vi "Multichannel Recording0.3.vi"() -> ()   [LabVIEW 2014]
uses:
  Enum State Typedef.ctl
  <vilib>/Utility/error.llb/DialogType.ctl
  <vilib>/_DAQmxBase/Internals/DAQmxBase Create Channel (AI-Voltage-Basic).vi
  <vilib>/_DAQmxBase/Internals/DAQmxBase Timing (Sample Clock).vi
  <vilib>/_DAQmxBase/Internals/DAQmxBase Read (Analog 2D DBL NChan NSamp).vi
panel:
  in  "Use Channel 0":bool caption="In Use?"
  in  "Use Channel 2":bool caption="In Use?"
  in  "Use Channel 3":bool caption="In Use?"
  in  "Use Channel 1":bool caption="In Use?"
  in  "Open Button":bool
  in  "Tab Control":T1(tab)
  in  "Amplifier Channel 0":T2 {"Amplifier Model" items=["Select a Model", "AM 1700", "BMA 200"]}
  out "Channel 0 Chart":waveform(dbl)(graph)
  in  "User Data Channel 0":T3
  out "Channel 1 Chart":waveform(dbl)(graph)
  in  "User Data Channel 1":T3
  in  "Amplifier Channel 1":T2 {"Amplifier Model" items=["Select a Model", "AM 1700", "BMA 200"]}
  out "Channel 2 Chart":waveform(dbl)(graph)
  in  "User Data Channel 2":T3
  in  "Amplifier Channel 2":T2 {"Amplifier Model" items=["Select a Model", "AM 1700", "BMA 200"]}
  out "Channel 3 Chart":waveform(dbl)(graph)
  in  "User Data Channel 3":T3
  in  "Amplifier Channel 3":T2 {"Amplifier Model" items=["Select a Model", "AM 1700", "BMA 200"]}
  out "Overview Chart":waveform(dbl)[](graph)
  in  "Stop Preview":bool
  in  "OK Button":bool
  out "State":T4
  in  "Clear Display":bool
  in  "Preview Button":bool
  out "Iterations Recorded":i32
  in  "Recording Time (seconds)":dbl
  in  "Sample Rate":i32=1000
  in  "Stop Button":bool
  out "Start Time hr/min":string
  out "Date mm/dd/yy":string
  in  "Exit Button":bool
  in  "Record Button":bool
  # "MSU EFISH Lab Multi-Channel Electronic Pulse Recorder"
  # "Must enter numbers into here before you start"
  # "Blue for On\nOrange for Off"
  # "DC"
  # "AC"
  # "Blue for AC and Orange for DC"
  # "Blue for On\nOrange for Off"
  # "DC"
  # "AC"
  # "Blue for AC and Orange for DC"
  # "Blue for On\nOrange for Off"
  # "DC"
  # "AC"
  # "Blue for AC and Orange for DC"
  # "Blue for On\nOrange for Off"
  # "DC"
  # "AC"
  # "Blue for AC and Orange for DC"
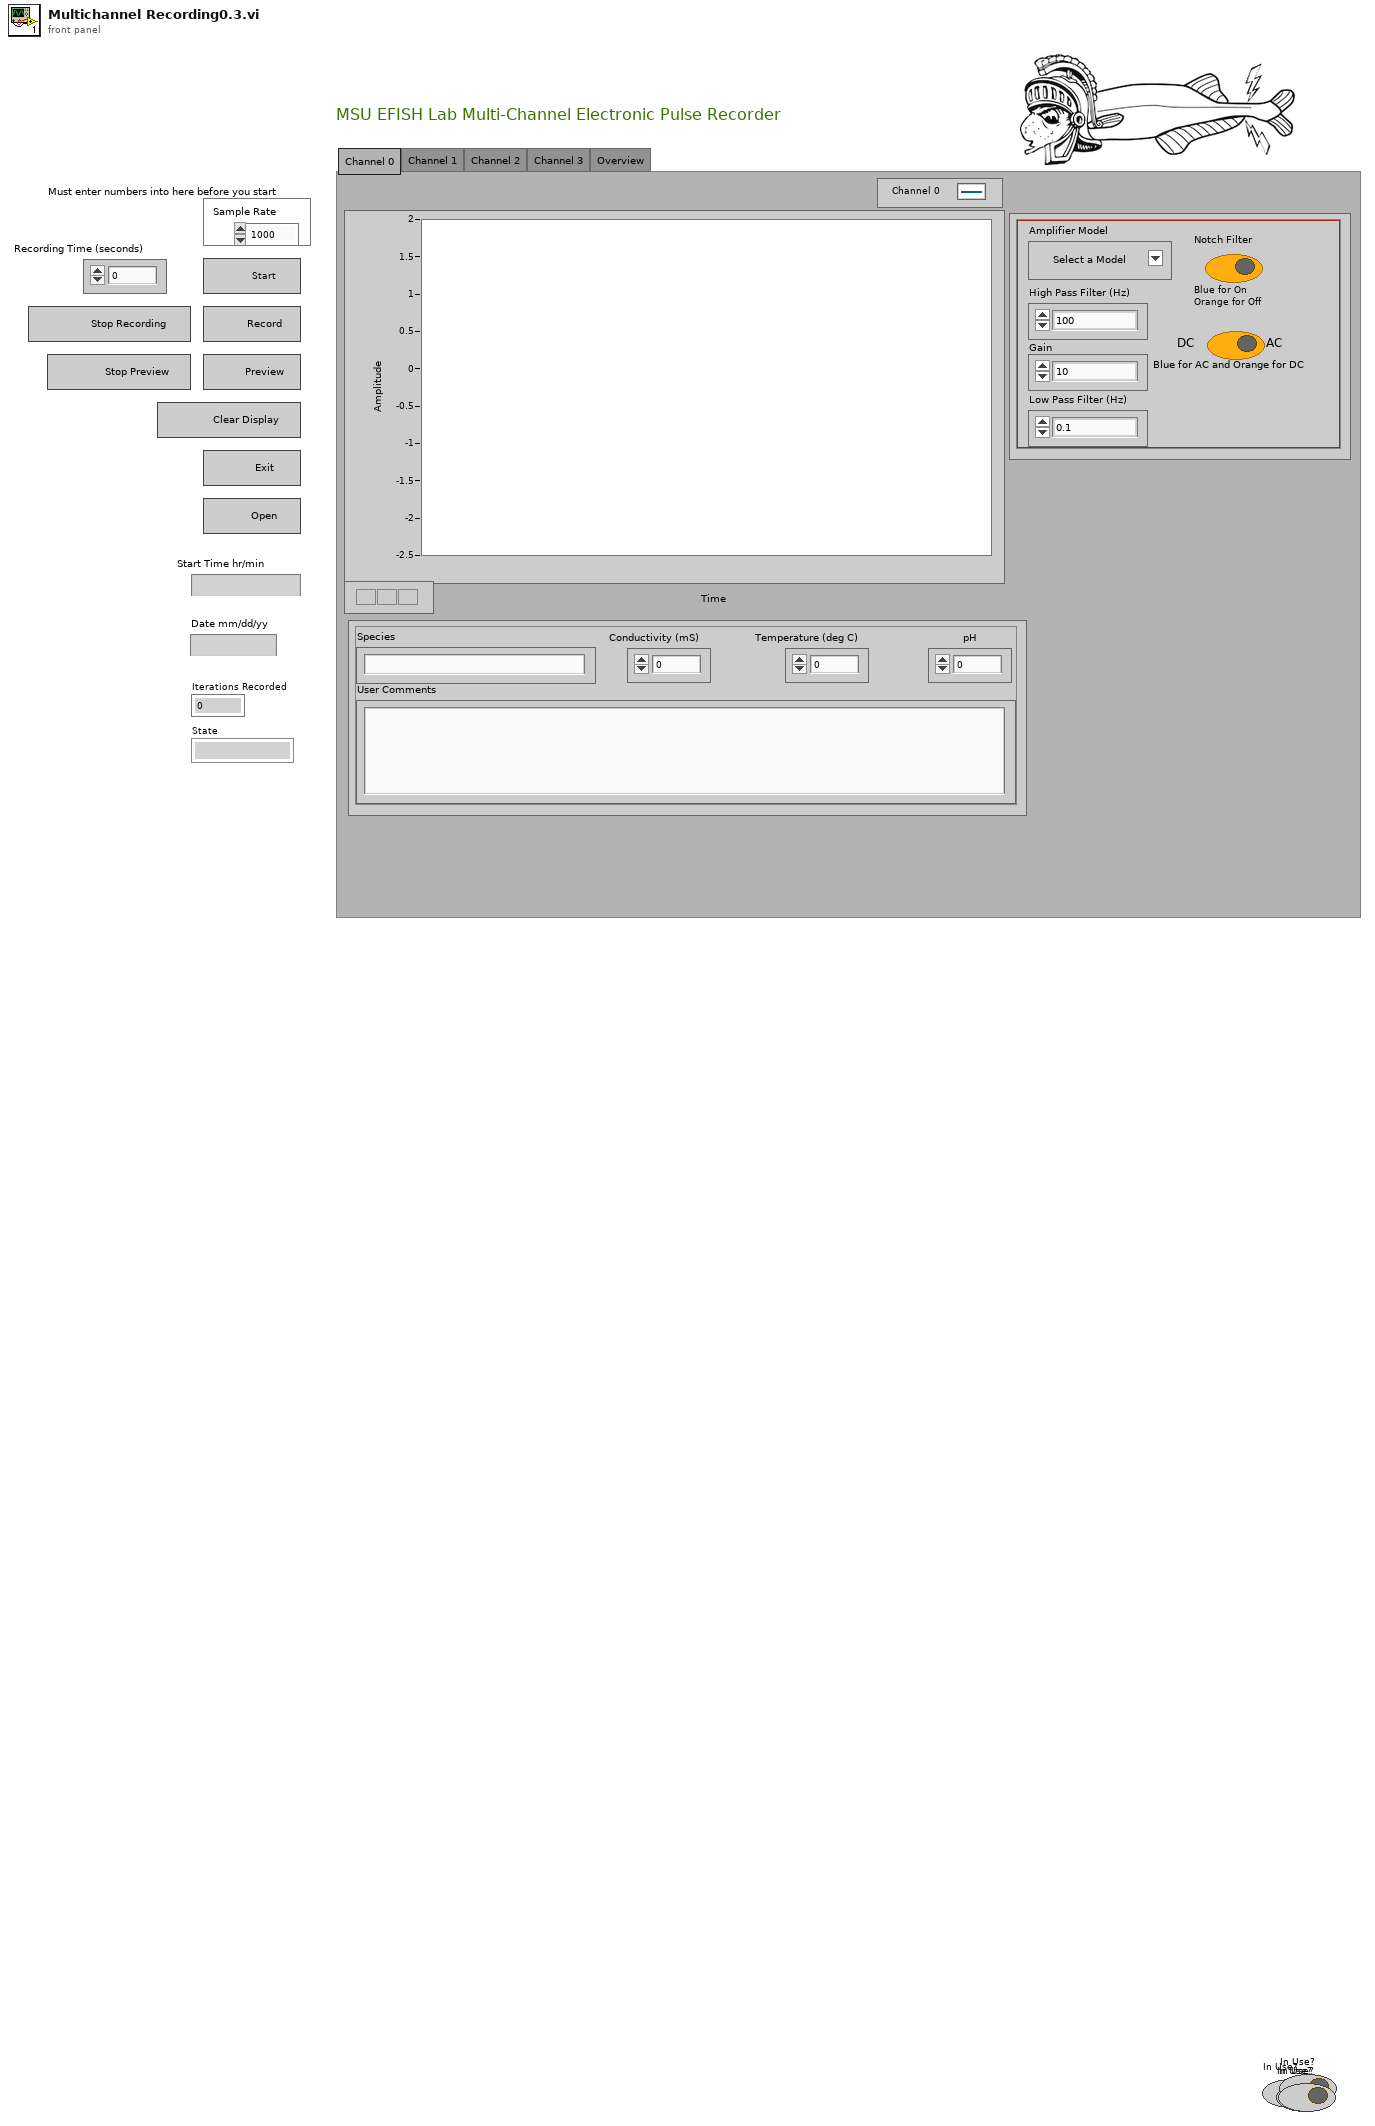
[diagram p1: front panel]
types:
  T1 = enum32{"Channel 0", "Channel 1", "Channel 2", "Channel 3", "Overview"}
  T2 = cluster{"Low Pass Filter (Hz)":enum16{"0.1", "1", "3", "10", "30", "100", "300"}, "Gain ":enum16{"10", "20", "50", "100", "200", "500", "1000", "2k", "5k", "10k", "20k", "50k"}, "High Pass Filter (Hz)":enum16{"100", "500", "1000", "3000", "5000", "10,000", "20,000", "30,000", "50,000"}, "Notch Filter":bool, "Amplifier Model":u16, "AC/DC Switch":bool}
  T3 = cluster{"pH":dbl, "Conductivity (mS)":dbl, "Temperature (deg C)":dbl, "User Comments":string, "Species":string}
  T4 = typedef "Enum State Typedef.ctl" = enum16{"", "Open FIle", "Beginning State", "Set the Sample Clock", "Prepreview Handling", "Clear Display", "Preview Data", "Stop", "Exit", "Record", "Create File"}
  T5 = cluster{"tdms file out":refnum<k34>, "tdms file out":refnum<k34>, "tdms file out":refnum<k34>, "tdms file out":refnum<k34>}
  T6 = enum8{"Enabled", "Disabled", "Disabled and Grayed Out"}
  T7 = typedef "DialogType.ctl" = u16
  T8 = enum16{"open", "open or create", "create or replace", "create", "open (read-only)"}
  T9 = cluster{"Use Channel 0":bool, "Use Channel 1":bool, "Use Channel 2":bool, "Use Channel 3":bool}
  T10 = cluster{"Waveform":waveform(dbl), "Waveform":waveform(dbl), "Waveform":waveform(dbl), "Waveform":waveform(dbl), waveform(dbl)[]}
  T11 = cluster{"Waveform":waveform(dbl), "Waveform":waveform(dbl), "Waveform":waveform(dbl), "Waveform":waveform(dbl)}
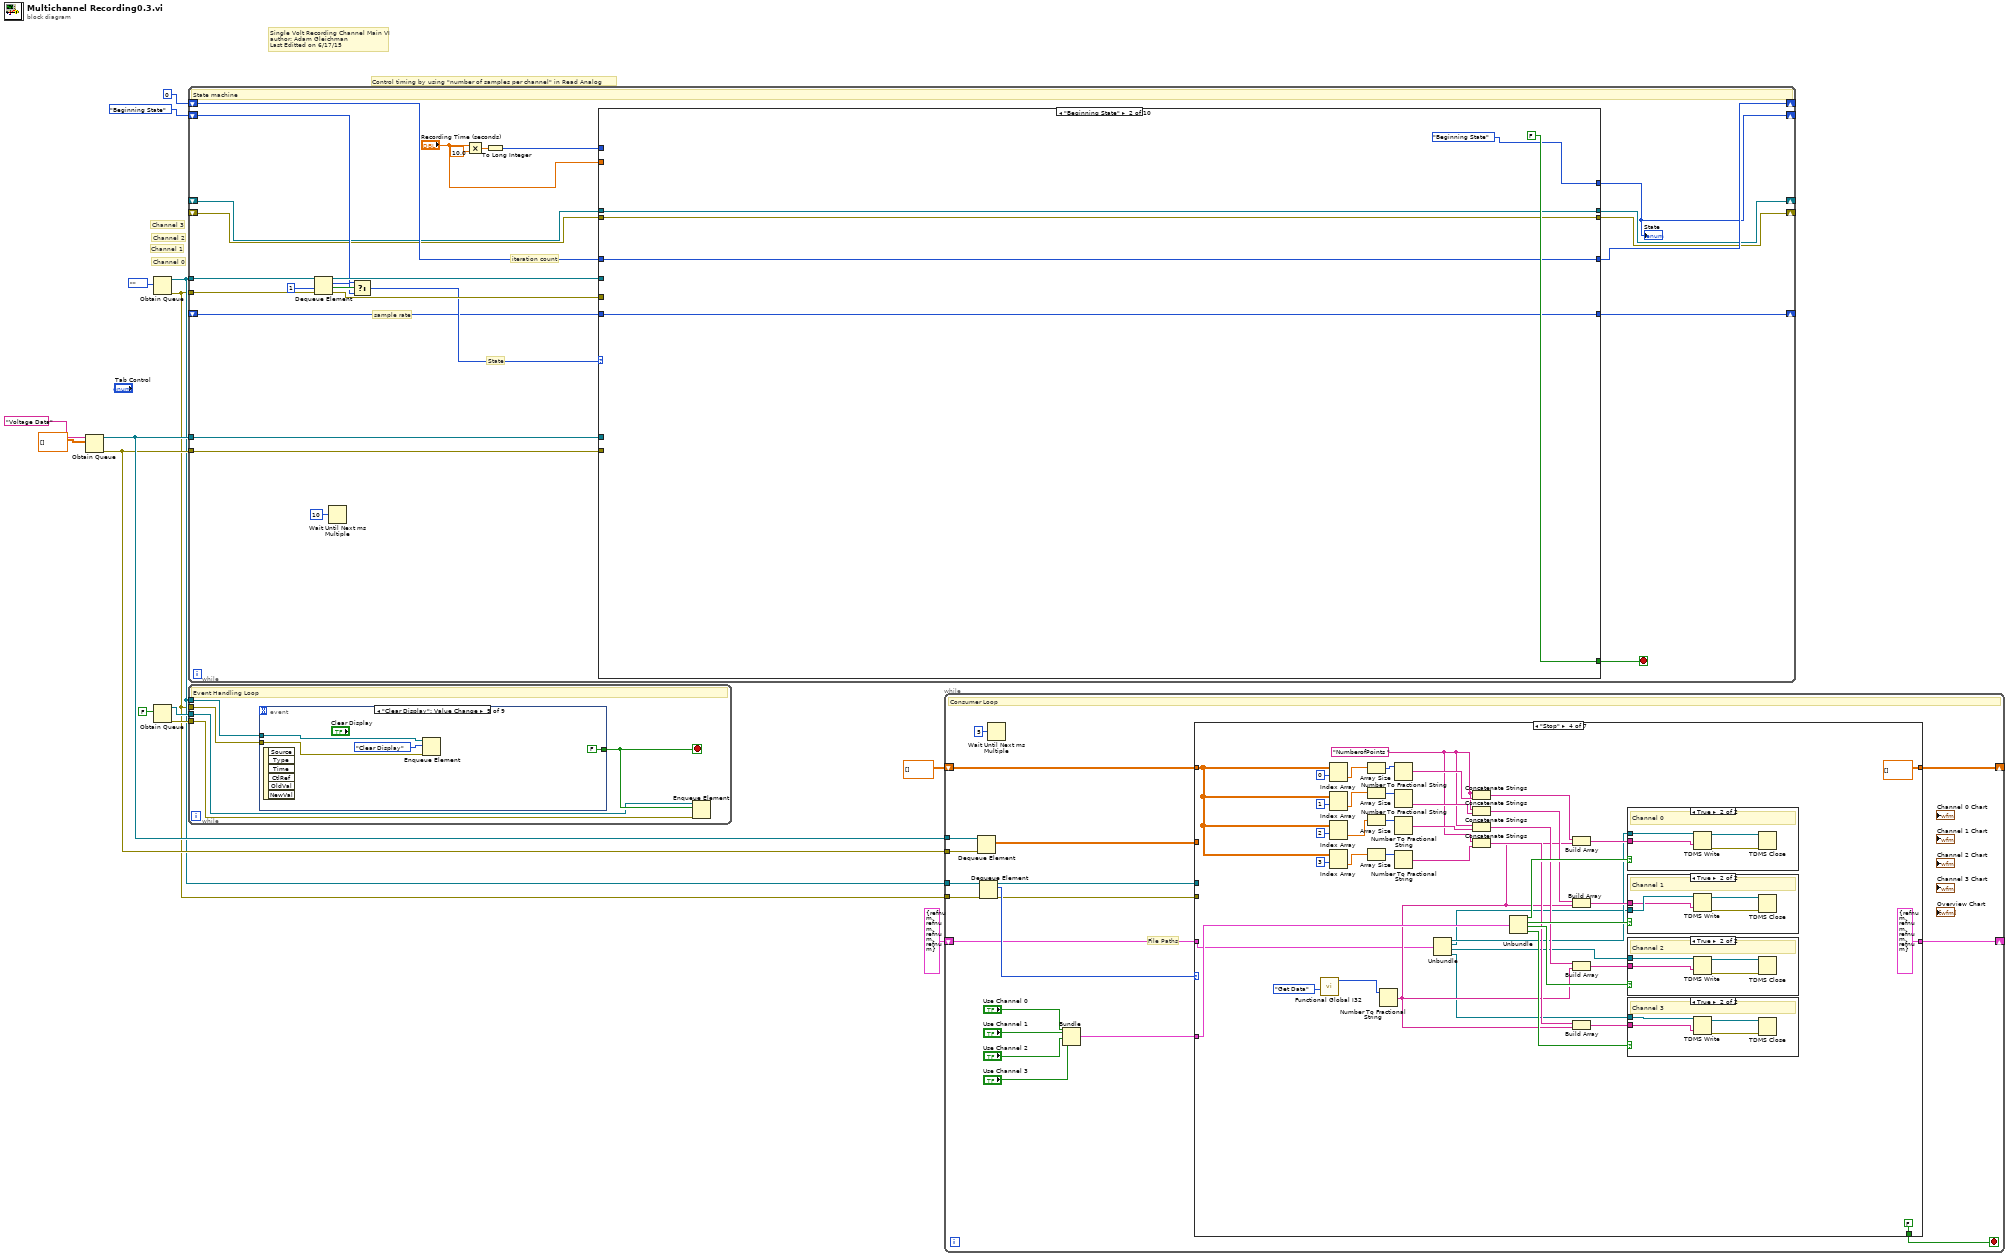
[diagram p0: block diagram]
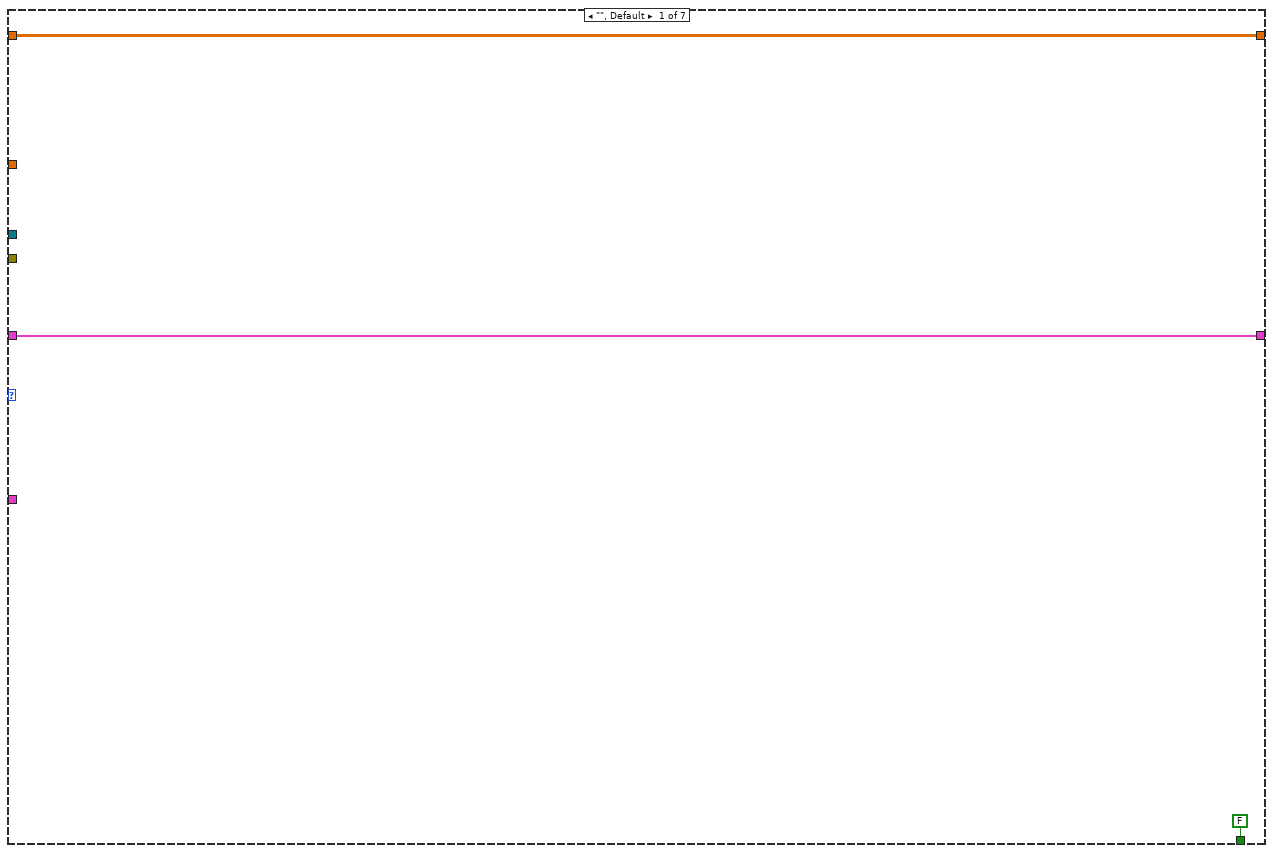
[diagram p2: hidden frame]
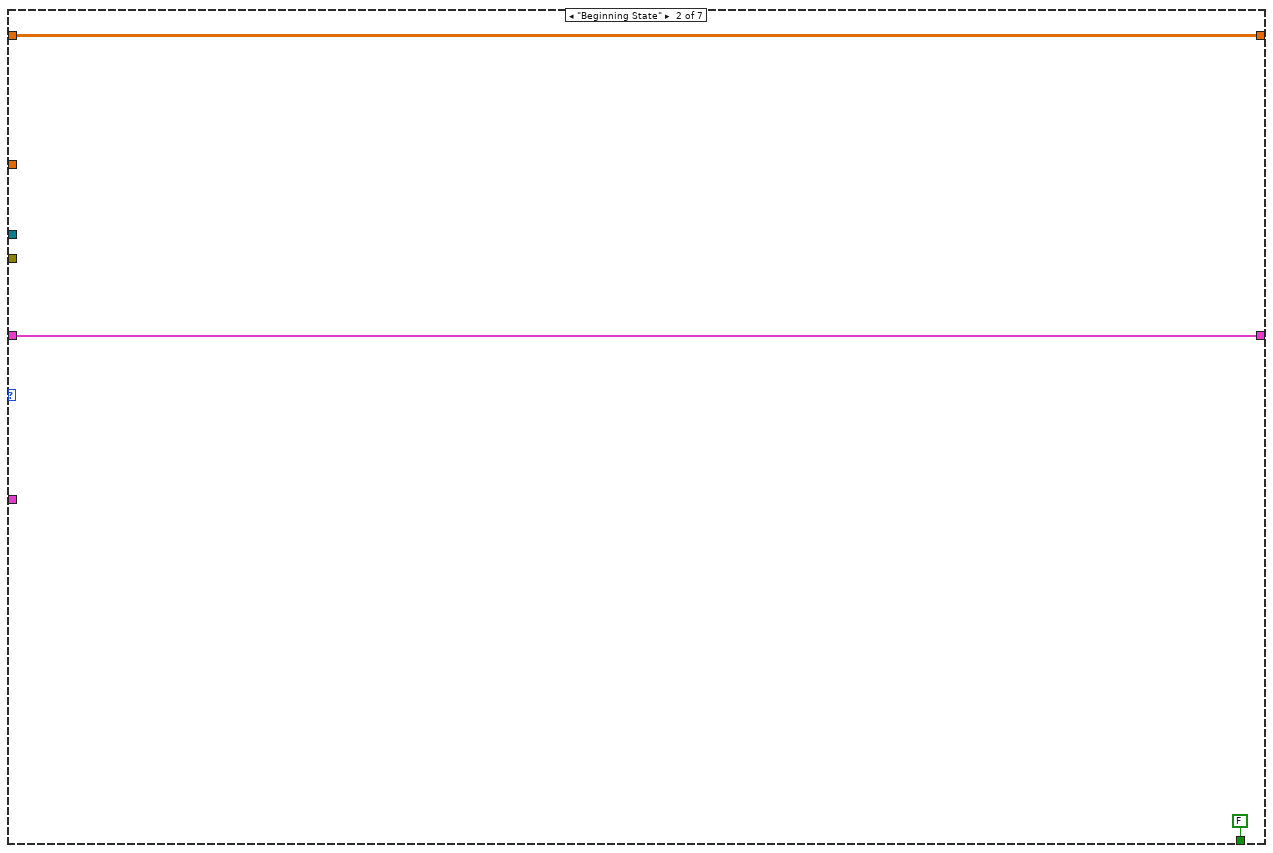
[diagram p3: hidden frame]
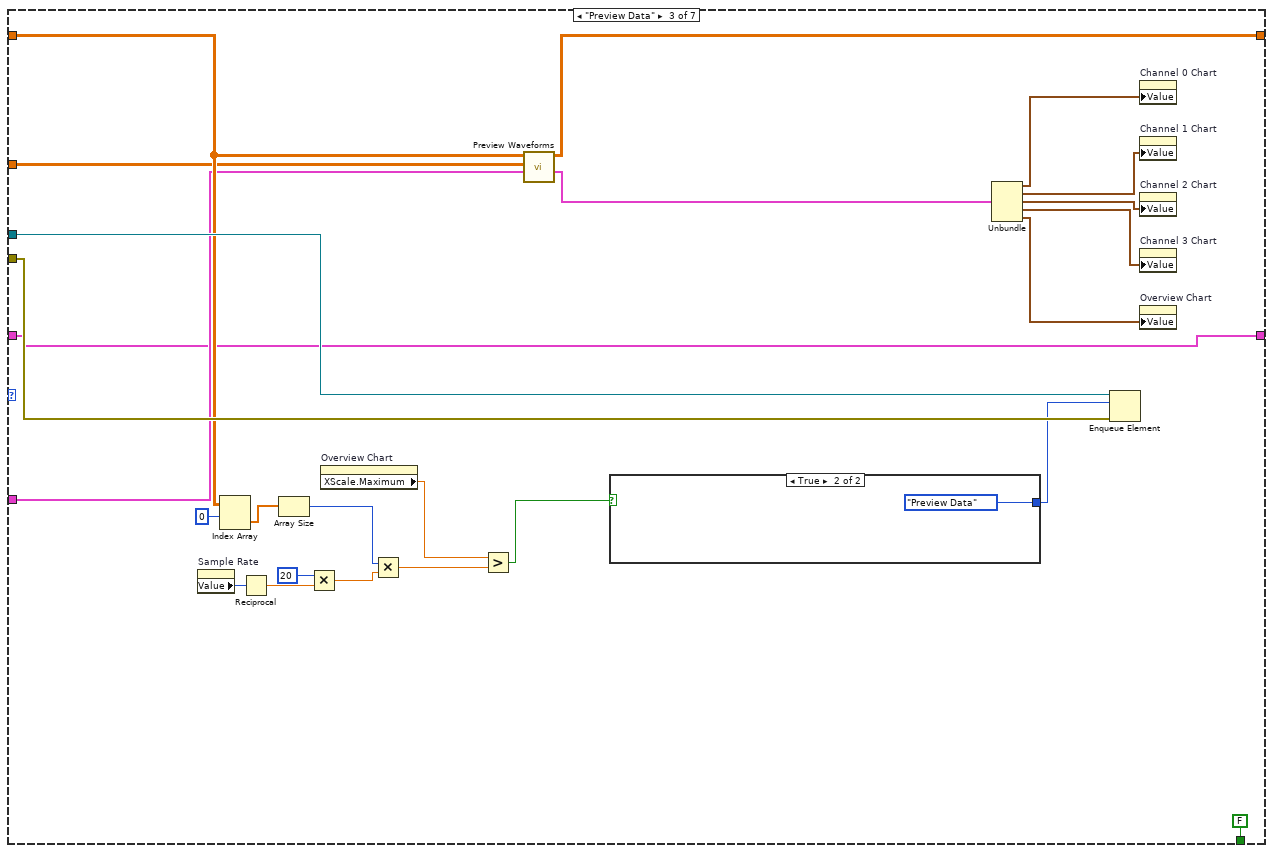
[diagram p4: hidden frame]
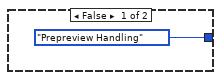
[diagram p5: hidden frame]
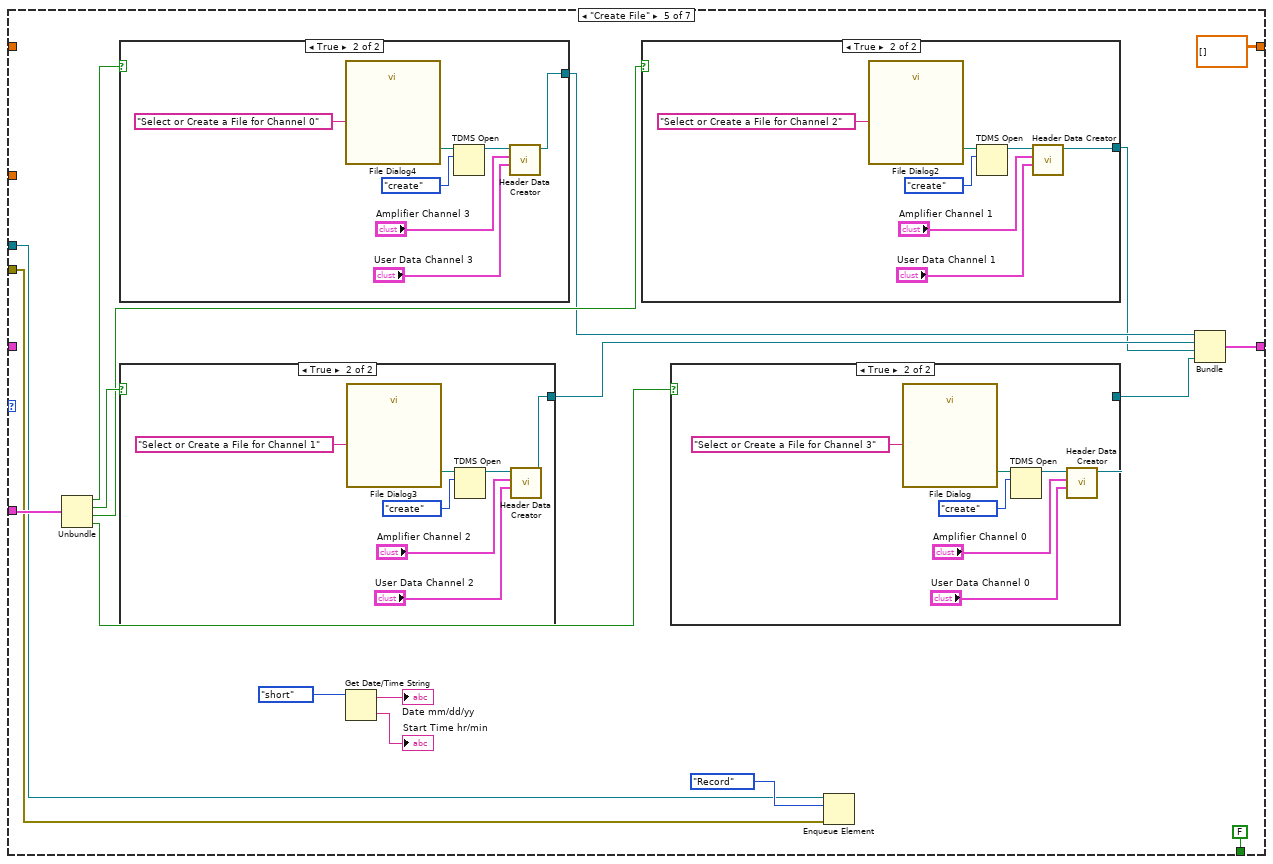
[diagram p10: hidden frame]
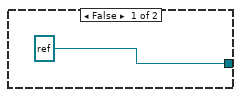
[diagram p11: hidden frame]
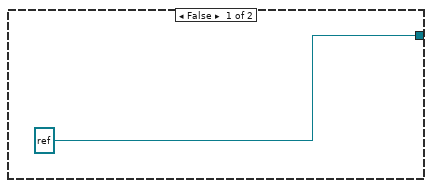
[diagram p12: hidden frame]
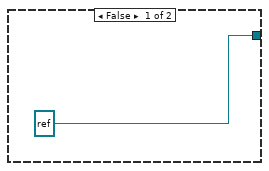
[diagram p13: hidden frame]
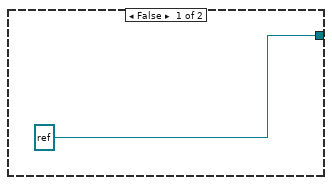
[diagram p14: hidden frame]
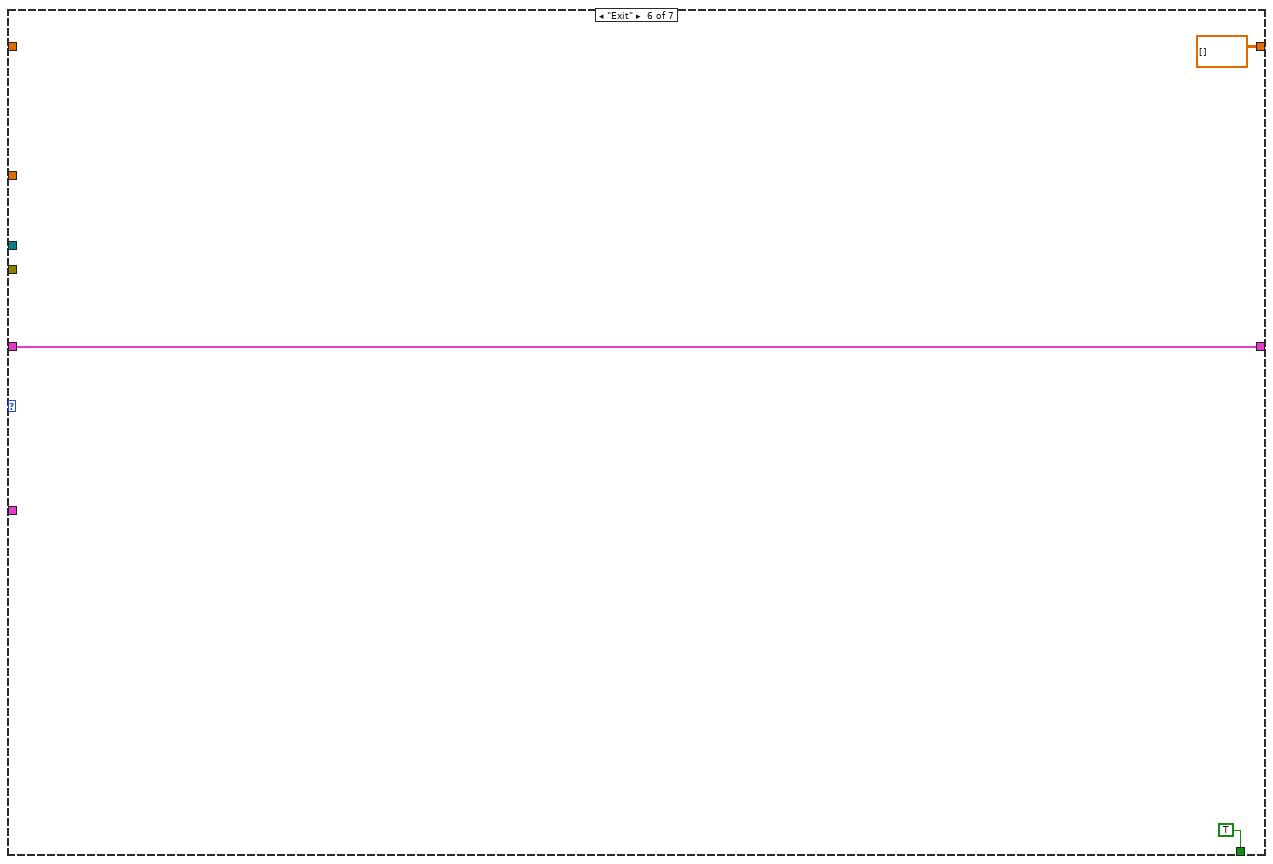
[diagram p15: hidden frame]
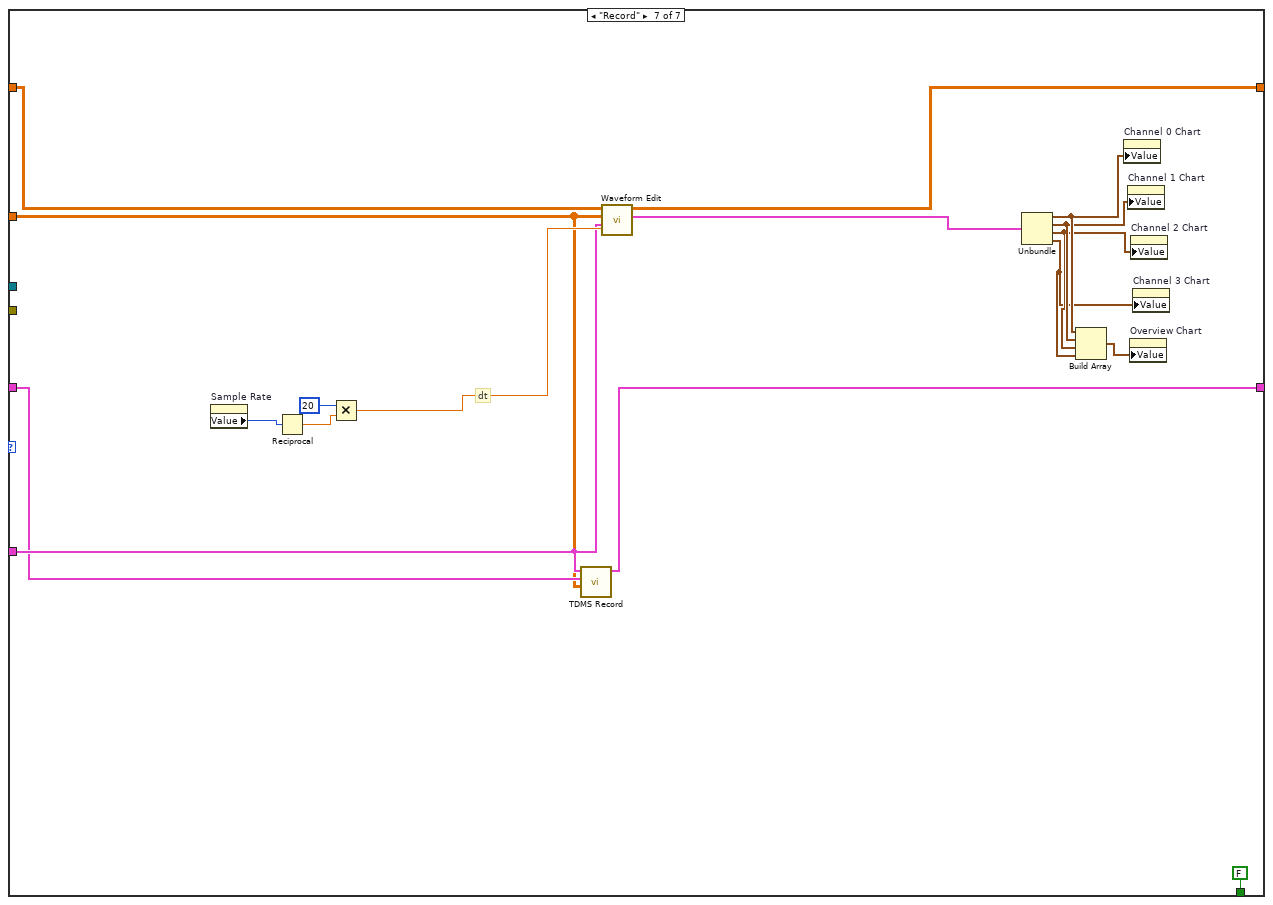
[diagram p16: hidden frame]
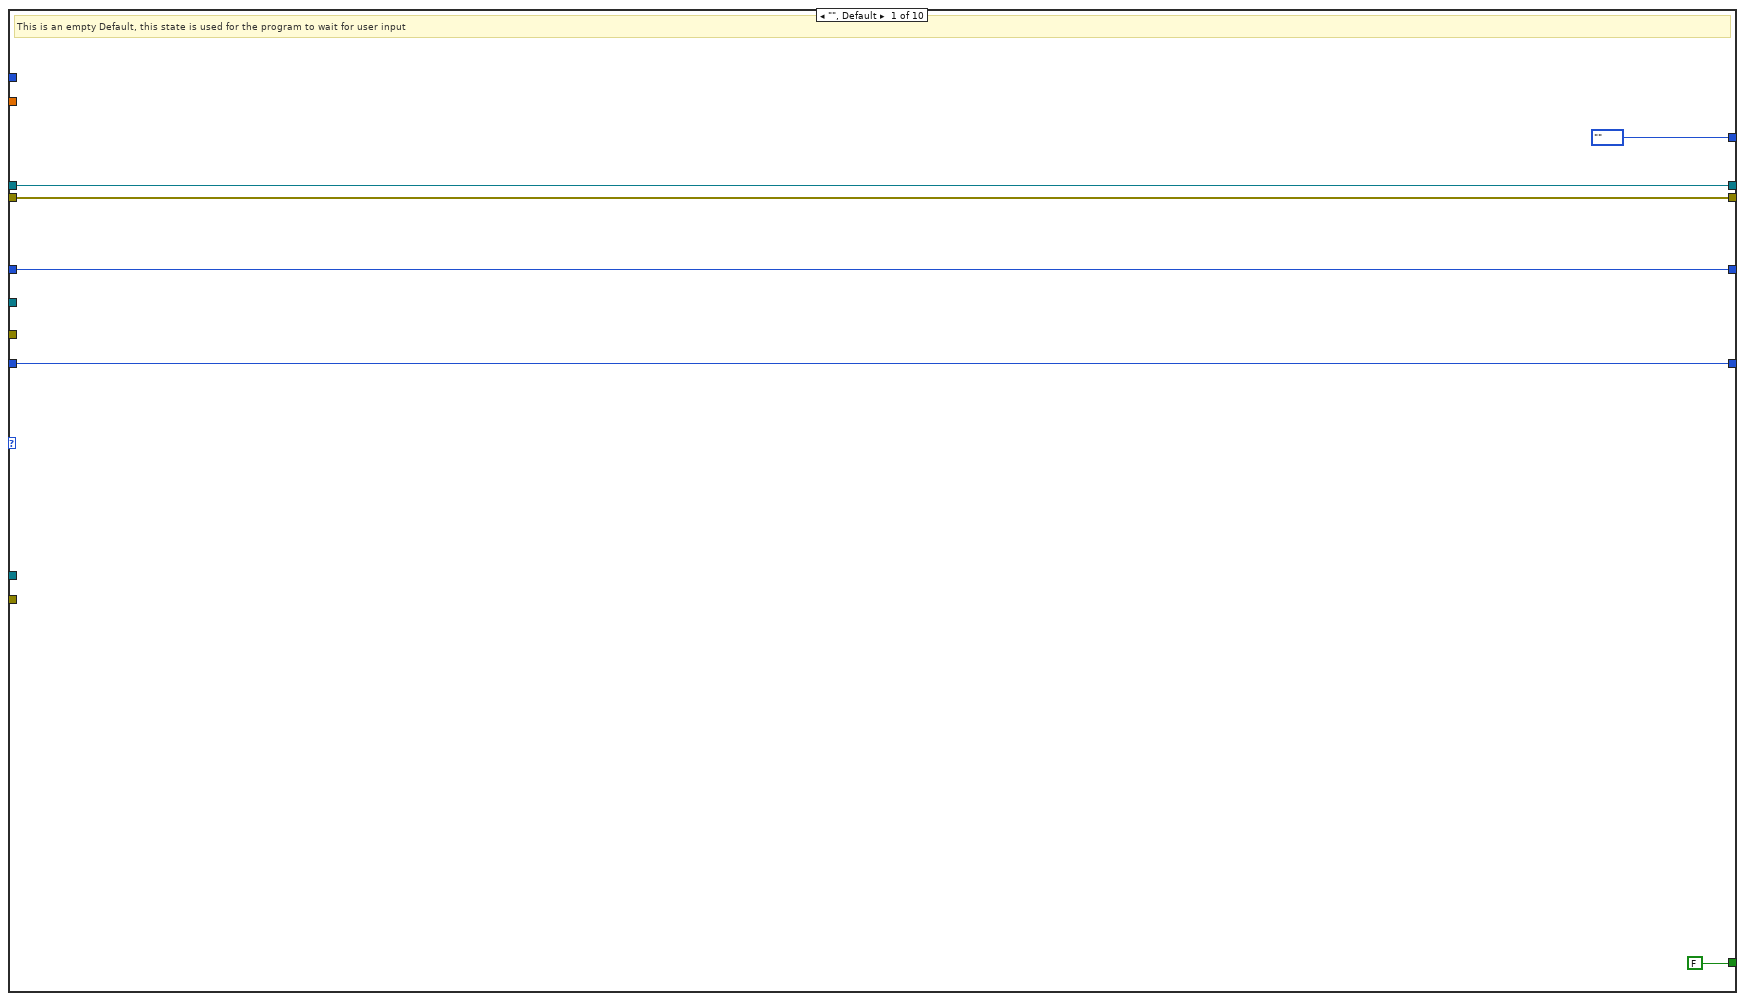
[diagram p17: hidden frame]
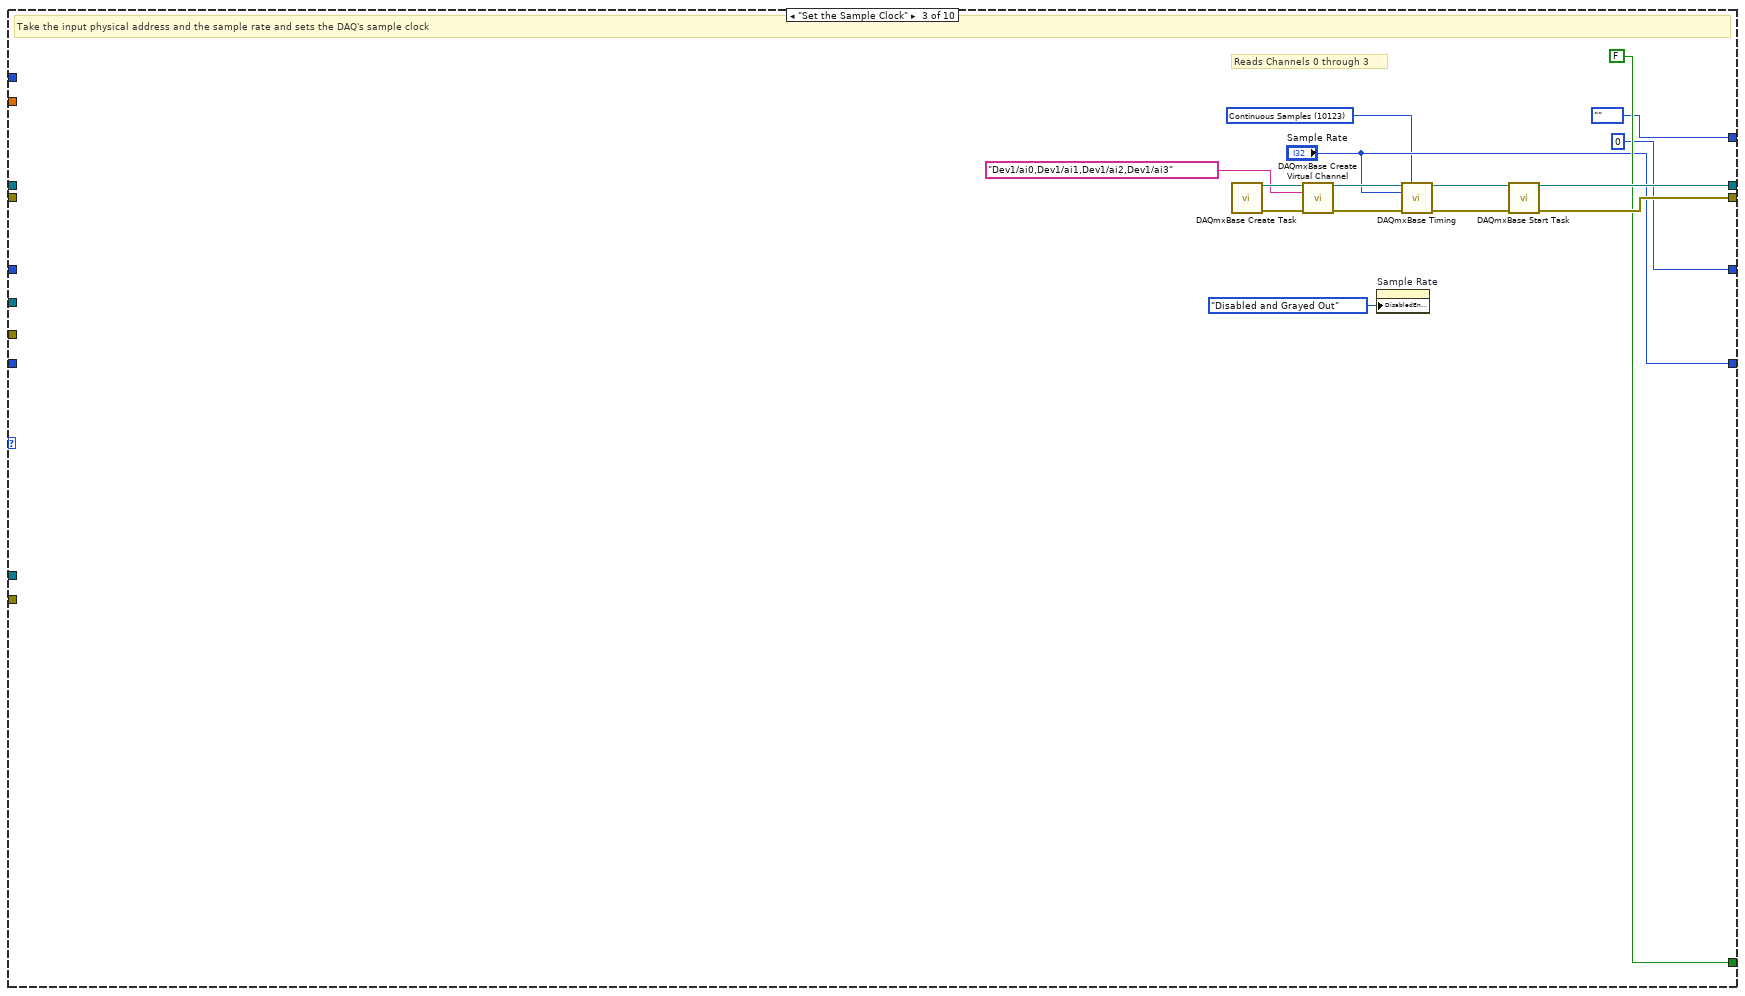
[diagram p18: hidden frame]
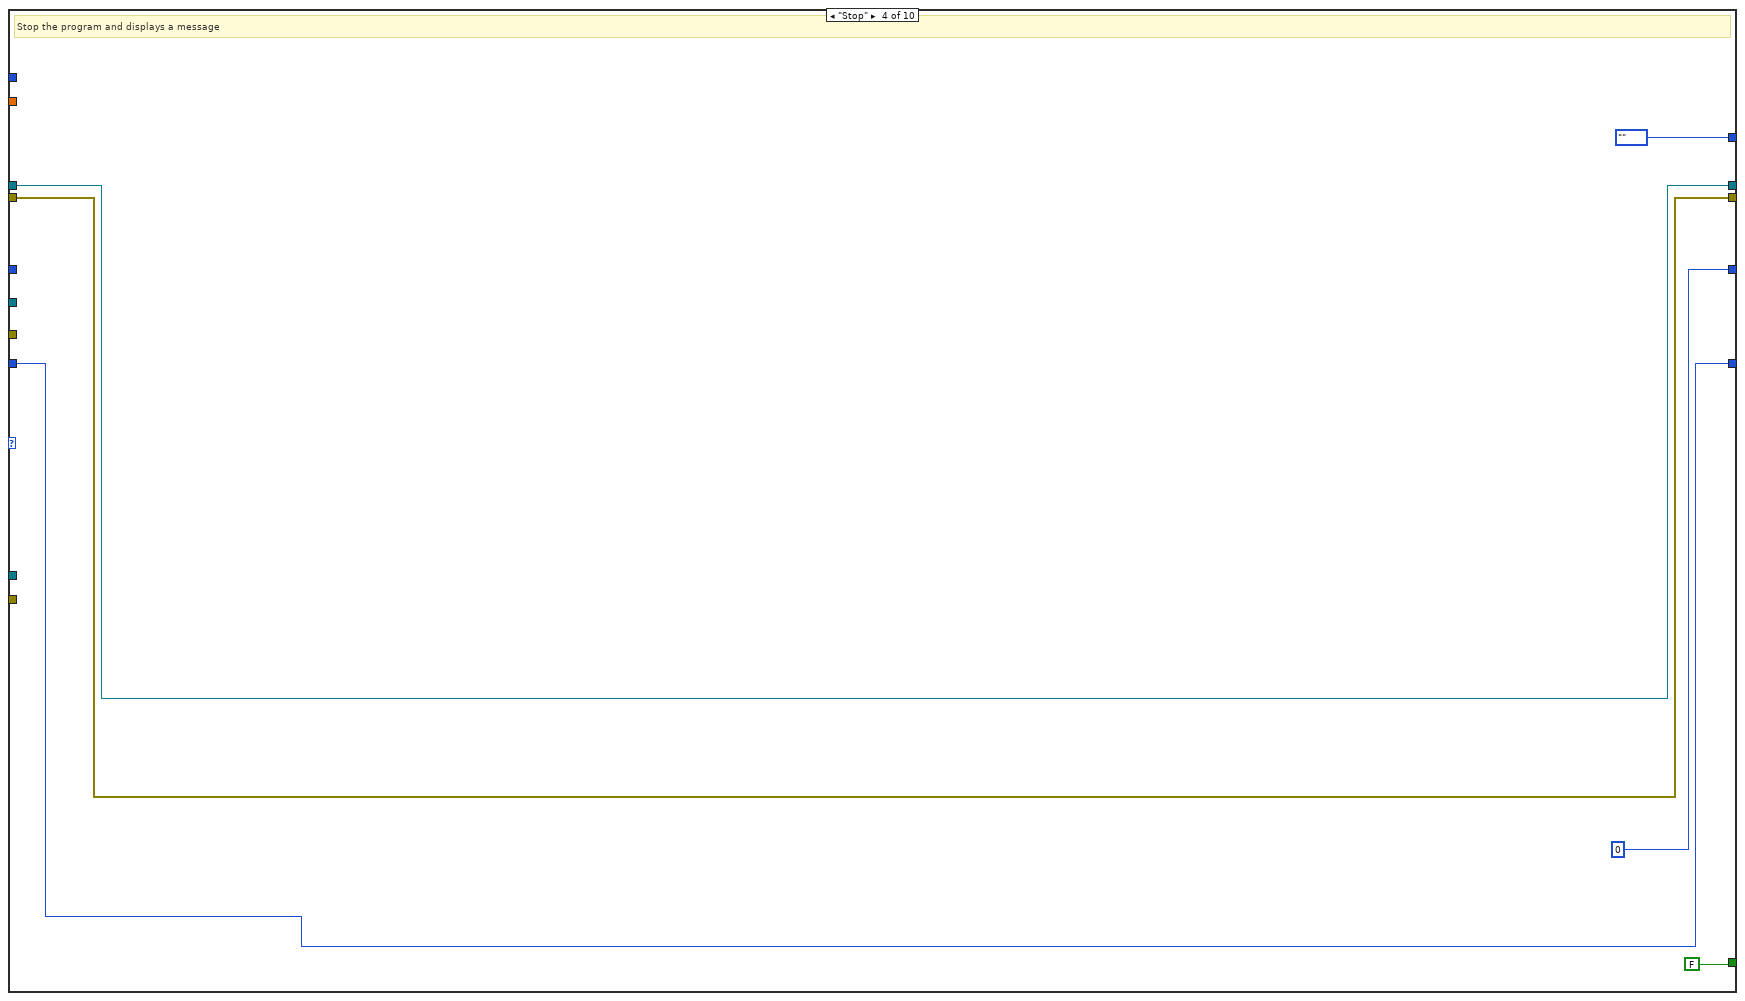
[diagram p19: hidden frame]
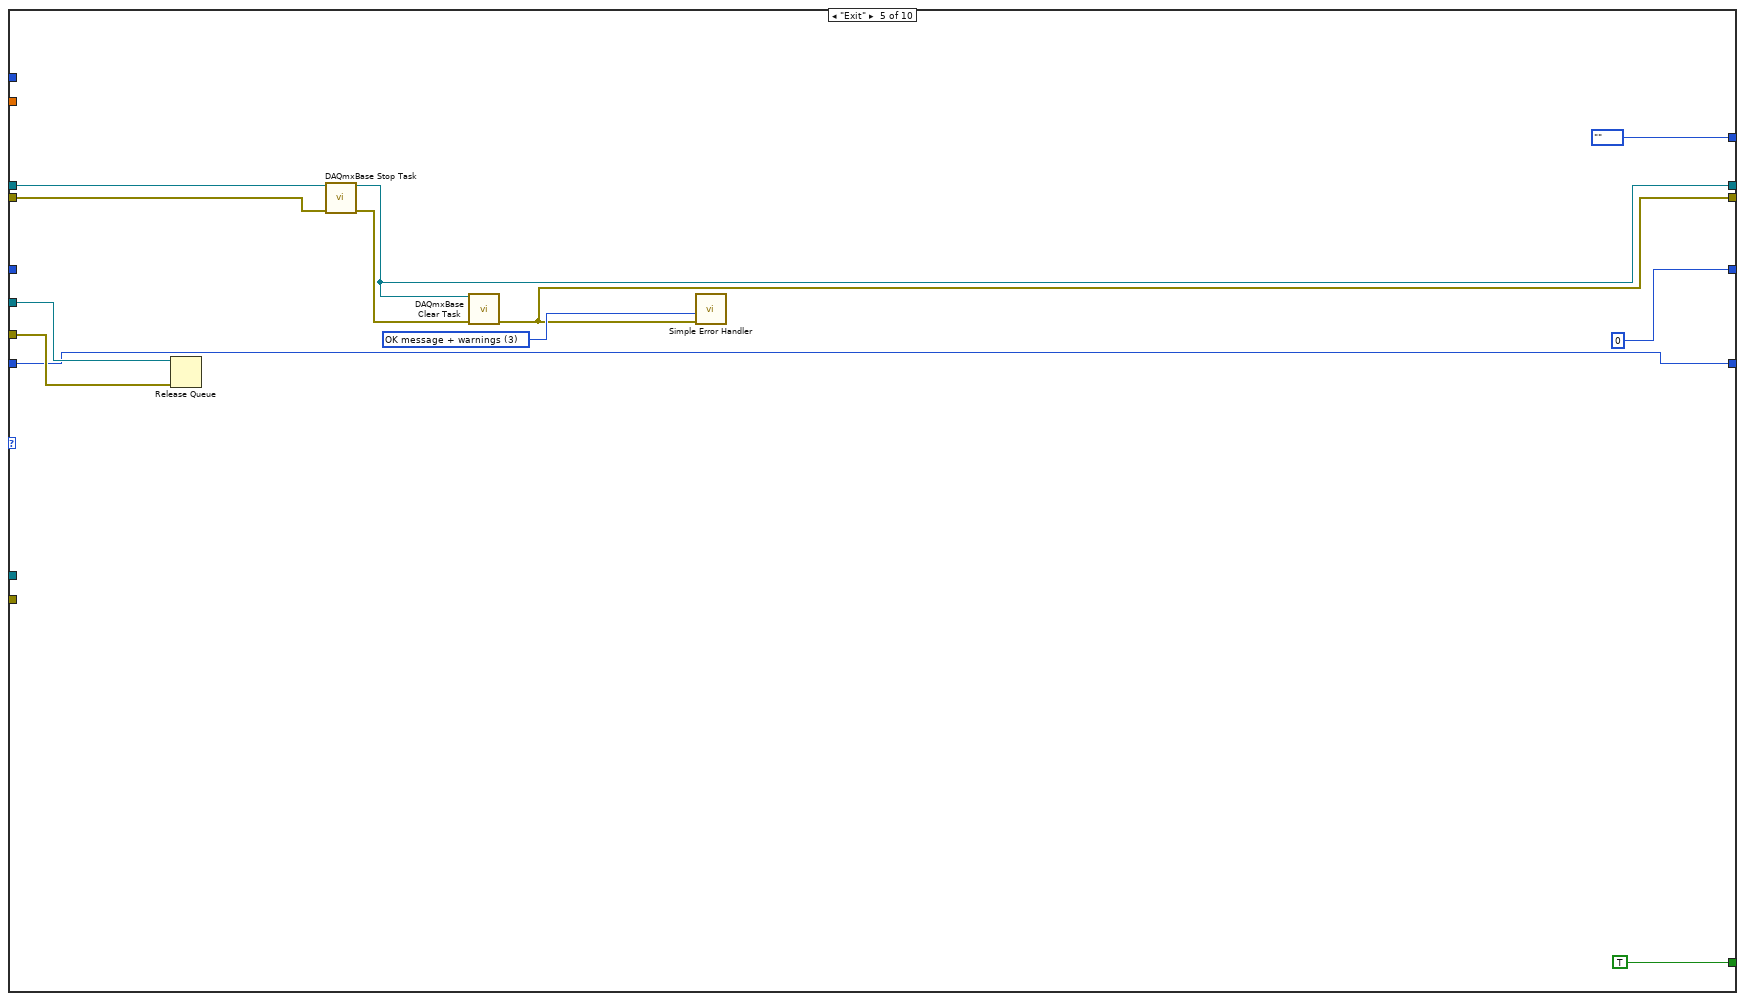
[diagram p20: hidden frame]
diagram:
  # "Channel 0"
  # "Channel 1"
  # "Channel 2"
  # "Channel 3"
  # "Single Volt Recording Channel Main VI\nauthor: Adam Gleichman\nLast Editted on 6/17/15"
  # "Control timing by using \"number of samples per channel\" in Read Analog"
  n1 = Obtain Queue(name (unnamed)="Voltage Data", element data type=dbl[][] []) -> (queue out=w6:refnum<queue>, error out=w5:errorcluster)  [unwired: 3 in, 1 out]
  n2 = Obtain Queue(element data type=FALSE) -> (queue out=w10:refnum<queue>, error out=w9:errorcluster)  [unwired: 4 in, 1 out]
  n3 = Obtain Queue(element data type=Enum_State_Typedef."" ("State")) -> (queue out=w4:refnum<queue>, error out=w3:errorcluster)  [unwired: 4 in, 1 out]
  n4 = while {
    tunnel: w4 -> [w40]
    tunnel: w3 -> [w39]
    shift-right: [w32] -> _
    shift-left: 0 -> [w33]
    shift-right: [w27] -> _
    shift-left: Enum_State_Typedef."Beginning State" ("State") -> [w29]
    shift-right: [w25] -> _
    shift-left: _ -> [w26]
    shift-right: [w21] -> _
    shift-left: _ -> [w19]
    shift-right: [w20] -> _
    shift-left: _ -> [w18]
    tunnel: w6 -> [w16]
    tunnel: w5 -> [w15]
    stop <- w38 stop-if-true
    # "State"
    # "iteration count"
    # "sample rate"
    # "State machine"
    n5 = Dequeue Element(queue=w40, timeout in ms (-1)=1, error in (no error)=w39) -> (queue out=w37:refnum<queue>, element=w30:T4, timed out?=w31:bool, error out=w36:errorcluster)
    n6 = Wait Until Next ms Multiple(millisecond multiple=u32 10) -> ()  [unwired: 1 out]
    n7 = Select(t=w29, s=w31, f=w30) -> (s? t:f=w28:T4)
    n8 = Multiply(x="Recording Time (seconds)", y=10.0) -> (x*y=w17:dbl)
    n9 = To Long Integer(number=w17) -> (32bit integer=w34:i32)
    n10 = case shown="\"Beginning State\"" w28 {
      tunnel: [FALSE FALSE FALSE FALSE TRUE FALSE FALSE FALSE FALSE FALSE] -> w38
      tunnel: w37 -> [_ _ _ _ w80 _ _ _ _ _]
      tunnel: w36 -> [_ _ _ _ w79 _ _ _ _ _]
      tunnel: w19 -> [w42 w50 _ w70 w83 w96 w114 w129 w139 w146]
      tunnel: w18 -> [w41 w51 _ w69 w82 w91 w113 w128 _ w145]
      tunnel: w26 -> [w43 w48 _ w68 w76 w86 w112 w127 w137 w147]
      tunnel: w34 -> [_ _ _ _ _ w103 _ _ _ _]
      tunnel: w33 -> [w45 w47 _ _ _ w104 w117 _ w138 w148]
      tunnel: [w45 w47 0 ("Sample Rate") 0 0 w98 w117 0 w138 w148] -> w32
      tunnel: [Enum_State_Typedef."" ("State") Enum_State_Typedef."Beginning State" ("State") Enum_State_Typedef."" ("State") Enum_State_Typedef."" ("State") Enum_State_Typedef."" ("State") w100 Enum_State_Typedef."" ("State") Enum_State_Typedef."Preview Data" ("State") Enum_State_Typedef."" ("State") Enum_State_Typedef."Preview Data" ("State")] -> w27
      tunnel: [w43 w48 "Sample Rate" w68 w76 w86 w112 w127 w137 w147] -> w25
      tunnel: "Recording Time (seconds)" -> [_ _ _ _ _ _ _ w122 _ _]
      tunnel: [w42 w50 w61 w70 w75 w96 w114 w129 w139 w146] -> w21
      tunnel: [w41 w51 w60 w69 w74 w90 w113 w128 w140 w145] -> w20
      tunnel: w16 -> [_ _ _ _ _ w89 _ w120 _ _]
      tunnel: w15 -> [_ _ _ _ _ w88 _ w119 _ _]
      frame "", Default {
        # "This is an empty Default, this state is used for the program to wait for user input"
      }
      frame "Beginning State" {
      }
      frame "Set the Sample Clock" {
        w54 = 10123 items=["Finite Samples"=10178, "Continuous Samples"=10123, "Hardware Timed Single Point"=12522] ("sample mode")
        # "Reads Channels 0 through 3"
        # "Take the input physical address and the sample rate and sets the DAQ's sample clock"
        n11 = call <vilib>:"DAQmxBase Create Task.vi"() -> ("task out"=w67:refnum<k21>, "error out"=w66:errorcluster)  [unwired: 14 in]
        n12 = call-poly <vilib>:"DAQmxBase Create Virtual Channel.vi"("task in"=w67, "physical channels"=tag "Dev1/ai0,Dev1/ai1,Dev1/ai2,Dev1/ai3", "error in"=w66) -> ("task out"=w65:refnum<k21>, "error out"=w64:errorcluster)  [unwired: 11 in]
        n13 = property on="Sample Rate" class="DigNum (strict)"("DisabledEnum"=T6."Disabled and Grayed Out" ("Disabled")) -> ()  [unwired: 2 in, 2 out]
        n14 = call-poly <vilib>:"DAQmxBase Timing.vi"("task/channels in"=w65, "sample mode"=w54, "rate"="Sample Rate", "error in"=w64) -> ("task out"=w63:refnum<k21>, "error out"=w62:errorcluster)  [unwired: 10 in]
        n15 = call <vilib>:"DAQmxBase Start Task.vi"("task/channels in"=w63, "error in"=w62) -> ("task out"=w61:refnum<k21>, "error out"=w60:errorcluster)  [unwired: 12 in]
      }
      frame "Stop" {
        # "Stop the program and displays a message"
      }
      frame "Exit" {
        w81 = T7 3 items=["no dialog", "OK message", "continue or stop message", "OK message + warnings", "continue/stop + warnings"] ("type of dialog (OK msg:1)")
        n16 = Release Queue(queue=w80, error in (no error)=w79) -> ()  [unwired: 1 in, 3 out]
        n17 = call <vilib>:"DAQmxBase Stop Task.vi"("task/channels in"=w83, "error in"=w82) -> ("task out"=w75:refnum<k21>, "error out"=w84:errorcluster)  [unwired: 12 in]
        n18 = call <vilib>:"DAQmxBase Clear Task.vi"("task in"=w75, "error in"=w84) -> ("error out"=w74:errorcluster)  [unwired: 13 in]
        n19 = call <vilib>:"Simple Error Handler.vi"("type of dialog (OK msg:1)"=w81, "error in (no error)"=w74) -> ()  [unwired: 3 in, 5 out]
      }
      frame "Record" {
        # "sample rate"
        # "Set the X Axis to Autoscale"
        n20 = property on="Channel 3 Chart" class="WFChart (strict)"("XScale.ScaleFit"=u8 2 ("X Scale.Scale Fit")) -> ()  [unwired: 2 in, 2 out]
        n21 = property on="Channel 0 Chart" class="WFChart (strict)"("XScale.ScaleFit"=u8 2 ("X Scale.Scale Fit")) -> ()  [unwired: 2 in, 2 out]
        n22 = property on="Channel 1 Chart" class="WFChart (strict)"("XScale.ScaleFit"=u8 2 ("X Scale.Scale Fit")) -> ()  [unwired: 2 in, 2 out]
        n23 = property on="Overview Chart" class="WFChart (strict)"("XScale.ScaleFit"=u8 2 ("X Scale.Scale Fit")) -> ()  [unwired: 2 in, 2 out]
        n24 = property on="Channel 2 Chart" class="WFChart (strict)"("XScale.ScaleFit"=u8 2 ("X Scale.Scale Fit")) -> ()  [unwired: 2 in, 2 out]
        n25 = Increment(x=w104) -> (x+1=w98:i32)
        "Iterations Recorded" <- w98
        n26 = Divide(x=w86, y=10) -> (x/y=w101:dbl)
        n27 = Greater Or Equal?(x=w98, y=w103) -> (x >= y?=w99:bool)
        n28 = call-poly <vilib>:"DAQmxBase Read.vi"("task/channels in"=w96, "number of samples per channel"=w101, "timeout"=100.0, "error in"=w91) -> ("data"=w87:dbl[][], "error out"=w90:errorcluster)  [unwired: 9 in, 1 out]
        n29 = case shown="True" w99 {
          tunnel: [Enum_State_Typedef."Record" ("State") Enum_State_Typedef."Stop" ("State")] -> w100
          frame False {
            # "Continue recording"
          }
          frame True {
            # "Finished recording"
            n30 = One Button Dialog(message="Recording is Finished") -> ()  [unwired: 1 in, 1 out]
          }
        }
        n31 = Enqueue Element(queue=w89, element=w87, error in (no error)=w88) -> ()  [unwired: 1 in, 3 out]
      }
      frame "Clear Display" {
        w110 = waveform(dbl)[] [] ("History Data")
        # "clears the data"
        # "Clears the graph"
        # "Clears the chart history"
        # "This clears the chart display"
        n32 = property on="Channel 0 Chart" class="WFChart (strict)"("History Data"=w110) -> ()  [unwired: 2 in, 2 out]
        n33 = property on="Channel 2 Chart" class="WFChart (strict)"("History Data"=w110) -> ()  [unwired: 2 in, 2 out]
        n34 = property on="Channel 1 Chart" class="WFChart (strict)"("History Data"=w110) -> ()  [unwired: 2 in, 2 out]
        n35 = property on="Channel 3 Chart" class="WFChart (strict)"("History Data"=w110) -> ()  [unwired: 2 in, 2 out]
        n36 = property on="Overview Chart" class="WFChart (strict)"("History Data"=waveform(dbl)[][] []) -> ()  [unwired: 2 in, 2 out]
      }
      frame "Preview Data" {
        # "This is not incrementing"
        # "Turns off the X auto scale"
        n37 = property on="Channel 0 Chart" class="WFChart (strict)"("XScale.ScaleFit"=u8 0 ("X Scale.Scale Fit")) -> ()  [unwired: 2 in, 2 out]
        n38 = property on="Channel 2 Chart" class="WFChart (strict)"("XScale.ScaleFit"=u8 0 ("X Scale.Scale Fit")) -> ()  [unwired: 2 in, 2 out]
        n39 = property on="Overview Chart" class="WFChart (strict)"("XScale.ScaleFit"=u8 0 ("X Scale.Scale Fit")) -> ()  [unwired: 2 in, 2 out]
        n40 = property on="Channel 3 Chart" class="WFChart (strict)"("XScale.ScaleFit"=u8 0 ("X Scale.Scale Fit")) -> ()  [unwired: 2 in, 2 out]
        n41 = property on="Channel 1 Chart" class="WFChart (strict)"("XScale.ScaleFit"=u8 0 ("X Scale.Scale Fit")) -> ()  [unwired: 2 in, 2 out]
        n42 = Divide(x=w127, y=10) -> (x/y=w131:dbl)
        n43 = property on="Overview Chart" class="WFChart (strict)"("XScale.Maximum"=w122) -> ()  [unwired: 2 in, 2 out]
        n44 = property on="Channel 0 Chart" class="WFChart (strict)"("XScale.Maximum"=w122) -> ()  [unwired: 2 in, 2 out]
        n45 = property on="Channel 1 Chart" class="WFChart (strict)"("XScale.Maximum"=w122) -> ()  [unwired: 2 in, 2 out]
        n46 = property on="Channel 2 Chart" class="WFChart (strict)"("XScale.Maximum"=w122) -> ()  [unwired: 2 in, 2 out]
        n47 = property on="Channel 3 Chart" class="WFChart (strict)"("XScale.Maximum"=w122) -> ()  [unwired: 2 in, 2 out]
        n48 = call-poly <vilib>:"DAQmxBase Read.vi"("task/channels in"=w129, "number of samples per channel"=w131, "timeout"=100.0, "error in"=w128) -> ("data"=w121:dbl[][])  [unwired: 9 in, 2 out]
        n49 = Enqueue Element(queue=w120, element=w121, error in (no error)=w119) -> ()  [unwired: 1 in, 3 out]
      }
      frame "Open FIle" {
        n50 = call "File Dialog5"() -> ("selected path"=w142:path)  [unwired: 12 in, 3 out]
        n51 = call <vilib>:"TDMS - File Viewer.vi"("file path"=w142) -> ("error out"=w140:errorcluster)  [unwired: 5 in, 1 out]
      }
      frame "Prepreview Handling" {
        w143 = waveform(dbl)[] [] ("History Data")
        # "This clears the Chart history"
        # "This clears the data before the preview data state starts"
        n52 = property on="Channel 2 Chart" class="WFChart (strict)"("History Data"=w143) -> ()  [unwired: 2 in, 2 out]
        n53 = property on="Channel 3 Chart" class="WFChart (strict)"("History Data"=w143) -> ()  [unwired: 2 in, 2 out]
        n54 = property on="Channel 1 Chart" class="WFChart (strict)"("History Data"=w143) -> ()  [unwired: 2 in, 2 out]
        n55 = property on="Channel 0 Chart" class="WFChart (strict)"("History Data"=w143) -> ()  [unwired: 2 in, 2 out]
        n56 = property on="Overview Chart" class="WFChart (strict)"("History Data"=waveform(dbl)[][] []) -> ()  [unwired: 2 in, 2 out]
      }
    }
    "State" <- w27
  }
  n57 = while {
    tunnel: w4 -> [w155]
    tunnel: w3 -> [w154]
    tunnel: w10 -> [w152]
    tunnel: w9 -> [w151]
    stop <- w153 stop-if-true
    # "Event Handling Loop"
    n58 = event shown="[8] \"Clear Display\": Value Change" {
      selector: _ -> [_ _ _ _ _ _ _ _ _]
      dyn-events: _ -> [_ _ _ _ _ _ _ _ _]
      timeout: _ -> [_ _ _ _ _ _ _ _ _]
      tunnel: [FALSE ("Exit Button") "Exit Button" FALSE ("Exit Button") FALSE ("Exit Button") FALSE ("Exit Button") FALSE ("Exit Button") FALSE ("Exit Button") FALSE ("Exit Button") FALSE ("Exit Button")] -> w153
      tunnel: w155 -> [_ w159 w164 w168 w172 w176 w180 w184 w188]
      tunnel: w154 -> [_ w158 w163 w167 w171 w175 w179 w183 w187]
      event Timeout {
        n59 = event-data() -> ()  [unwired: 1 in, 3 out]
      }
      event "Exit Button": Value Change {
        n60 = event-data() -> ()  [unwired: 1 in, 1 out]
        n61 = Enqueue Element(queue=w159, element=Enum_State_Typedef."Exit", error in (no error)=w158) -> ()  [unwired: 1 in, 3 out]
      }
      event "Preview Button": Value Change {
        n62 = event-data() -> ()  [unwired: 1 in, 6 out]
        n63 = Enqueue Element(queue=w164, element=Enum_State_Typedef."Preview Data", error in (no error)=w163) -> ()  [unwired: 1 in, 3 out]
      }
      event "Stop Preview": Value Change {
        n64 = event-data() -> ()  [unwired: 1 in, 6 out]
        n65 = Enqueue Element(queue=w168, element=Enum_State_Typedef."", error in (no error)=w167) -> ()  [unwired: 1 in, 3 out]
      }
      event "Open Button": Value Change {
        n66 = event-data() -> ()  [unwired: 1 in, 6 out]
        n67 = Enqueue Element(queue=w172, element=Enum_State_Typedef."Open FIle", error in (no error)=w171) -> ()  [unwired: 1 in, 3 out]
      }
      event "OK Button": Value Change {
        n68 = event-data() -> ()  [unwired: 1 in, 6 out]
        n69 = Enqueue Element(queue=w176, element=Enum_State_Typedef."Set the Sample Clock", error in (no error)=w175) -> ()  [unwired: 1 in, 3 out]
      }
      event "Stop Button": Value Change {
        n70 = event-data() -> ()  [unwired: 1 in, 6 out]
        n71 = Enqueue Element(queue=w180, element=Enum_State_Typedef."Stop", error in (no error)=w179) -> ()  [unwired: 1 in, 3 out]
      }
      event "Record Button": Value Change {
        n72 = event-data() -> ()  [unwired: 1 in, 6 out]
        n73 = Enqueue Element(queue=w184, element=Enum_State_Typedef."Create File", error in (no error)=w183) -> ()  [unwired: 1 in, 3 out]
      }
      event "Clear Display": Value Change {
        n74 = event-data() -> ()  [unwired: 1 in, 6 out]
        n75 = Enqueue Element(queue=w188, element=Enum_State_Typedef."Clear Display", error in (no error)=w187) -> ()  [unwired: 1 in, 3 out]
      }
    }
    n76 = Enqueue Element(queue=w152, element=w153, error in (no error)=w151) -> ()  [unwired: 1 in, 3 out]
  }
  n77 = while {
    tunnel: w6 -> [w207]
    tunnel: w5 -> [w206]
    tunnel: w4 -> [w200]
    tunnel: w3 -> [w199]
    shift-right: [w191] -> _
    shift-left: dbl[][] [] -> [w195]
    shift-right: [w193] -> _
    shift-left: T5 {"tdms file out"=refnum, "tdms file out"=refnum, "tdms file out"=refnum, "tdms file out"=refnum} ("Output TDMS File Cluster") -> [w189]
    stop <- w190 stop-if-true
    # "File Paths"
    # "Consumer Loop"
    n78 = Dequeue Element(queue=w207, error in (no error)=w206) -> (element=w192:dbl[][])  [unwired: 1 in, 3 out]
    n79 = Dequeue Element(queue=w200, error in (no error)=w199) -> (queue out=w197:refnum<queue>, element=w198:T4, error out=w196:errorcluster)  [unwired: 1 in, 1 out]
    n80 = Wait Until Next ms Multiple(millisecond multiple=u32 5) -> ()  [unwired: 1 out]
    n81 = Bundle("Use Channel 0"="Use Channel 0", "Use Channel 1"="Use Channel 1", "Use Channel 2"="Use Channel 2", "Use Channel 3"="Use Channel 3") -> (w194:T9)  [unwired: 1 in]
    n82 = case shown="\"Stop\"" w198 {
      tunnel: w197 -> [_ _ w238 _ w302 _ _]
      tunnel: w196 -> [_ _ w237 _ w301 _ _]
      tunnel: w195 -> [w209 w213 w233 w272 _ _ w366]
      tunnel: w194 -> [_ _ w231 w270 w313 _ w355]
      tunnel: [w208 w212 w214 T5 {"tdms file out"=refnum, "tdms file out"=refnum, "tdms file out"=refnum, "tdms file out"=refnum} ("Output TDMS File Cluster") w304 w349 w352] -> w193
      tunnel: w192 -> [_ _ w232 _ _ _ w353]
      tunnel: [w209 w213 w230 dbl[][] [] ("Output Decimated Data") dbl[][] [] ("Output Decimated Data") dbl[][] [] ("Output Decimated Data") w365] -> w191
      tunnel: [FALSE FALSE FALSE FALSE FALSE TRUE FALSE] -> w190
      tunnel: w189 -> [w208 w212 w214 w248 _ w349 w354]
      frame "", Default {
      }
      frame "Beginning State" {
      }
      frame "Preview Data" {
        n83 = property on="Sample Rate" class="DigNum (strict)"() -> ("Value"=w223:i32)  [unwired: 2 in, 2 out]
        n84 = Index Array(array=w233, index (row)=0) -> (element=w234:dbl[])  [unwired: 1 in]
        n85 = Reciprocal(x=w223) -> (1/x=w222:dbl)
        n86 = Array Size(array=w234) -> (size(s)=w219:i32)
        n87 = Multiply(x=u16 20, y=w222) -> (x*y=w220:dbl)
        n88 = property on="Overview Chart" class="WFChart (strict)"() -> ("XScale.Maximum"=w217:dbl)  [unwired: 2 in, 2 out]
        n89 = Multiply(x=w219, y=w220) -> (x*y=w218:dbl)
        n90 = Greater?(x=w217, y=w218) -> (0:w216:bool)
        n91 = call "Preview Waveforms.vi"("In Use Cluster"=w231, "Input Read Data"=w232, "Input Decimated Data"=w233) -> ("Output Waveform Cluster"=w229:T10, "Output Data"=w230:dbl[][])  [unwired: 7 in]
        n92 = case shown="True" w216 {
          tunnel: [Enum_State_Typedef."Prepreview Handling" ("State") Enum_State_Typedef."Preview Data" ("State")] -> w236
          frame False {
          }
          frame True {
          }
        }
        n93 = Unbundle(w229) -> ("Waveform"=w228:waveform(dbl), "Waveform"=w227:waveform(dbl), "Waveform"=w226:waveform(dbl), "Waveform"=w224:waveform(dbl), w225:waveform(dbl)[])
        n94 = Enqueue Element(queue=w238, element=w236, error in (no error)=w237) -> ()  [unwired: 1 in, 3 out]
        n95 = property on="Channel 0 Chart" class="WFChart (strict)"("Value"=w228) -> ()  [unwired: 2 in, 2 out]
        n96 = property on="Channel 1 Chart" class="WFChart (strict)"("Value"=w227) -> ()  [unwired: 2 in, 2 out]
        n97 = property on="Channel 2 Chart" class="WFChart (strict)"("Value"=w226) -> ()  [unwired: 2 in, 2 out]
        n98 = property on="Channel 3 Chart" class="WFChart (strict)"("Value"=w224) -> ()  [unwired: 2 in, 2 out]
        n99 = property on="Overview Chart" class="WFChart (strict)"("Value"=w225) -> ()  [unwired: 2 in, 2 out]
      }
      frame "Stop" {
        w261 = "NumberofPoints " ("string")
        n100 = call "Functional Global I32.vi"("Enum"=enum16{"Set Data", "Get Data"}."Get Data") -> ("Integer"=w254:i32)  [unwired: 10 in]
        n101 = Index Array(array=w272, index (row)=0) -> (element=w279:dbl[])  [unwired: 1 in]
        n102 = Index Array(array=w272, index (row)=1) -> (element=w280:dbl[])  [unwired: 1 in]
        n103 = Index Array(array=w272, index (row)=2) -> (element=w278:dbl[])  [unwired: 1 in]
        n104 = Index Array(array=w272, index (row)=3) -> (element=w277:dbl[])  [unwired: 1 in]
        n105 = Array Size(array=w279) -> (size(s)=w282:i32)
        n106 = Array Size(array=w280) -> (size(s)=w281:i32)
        n107 = Array Size(array=w278) -> (size(s)=w263:i32)
        n108 = Array Size(array=w277) -> (size(s)=w262:i32)
        n109 = Number To Fractional String(number=w254) -> (F-format string=w253:string)  [unwired: 3 in]
        n110 = Number To Fractional String(number=w282) -> (F-format string=w271:string)  [unwired: 3 in]
        n111 = Number To Fractional String(number=w281) -> (F-format string=w265:string)  [unwired: 3 in]
        n112 = Number To Fractional String(number=w263) -> (F-format string=w264:string)  [unwired: 3 in]
        n113 = Number To Fractional String(number=w262) -> (F-format string=w260:string)  [unwired: 3 in]
        n114 = Unbundle(w248) -> ("tdms file out"=w247:refnum<k34>, "tdms file out"=w246:refnum<k34>, "tdms file out"=w245:refnum<k34>, "tdms file out"=w244:refnum<k34>)
        n115 = Concatenate Strings(w261, w271) -> (w259:string)
        n116 = Concatenate Strings(w261, w265) -> (w258:string)
        n117 = Concatenate Strings(w261, w264) -> (w257:string)
        n118 = Concatenate Strings(w261, w260) -> (w256:string)
        n119 = Unbundle(w270) -> ("Use Channel 0"=w269:bool, "Use Channel 1"=w268:bool, "Use Channel 2"=w267:bool, "Use Channel 3"=w266:bool)
        n120 = Build Array(w259, w253) -> (w249:string[])
        n121 = Build Array(w258, w253) -> (w250:string[])
        n122 = Build Array(w257, w253) -> (w251:string[])
        n123 = Build Array(w256, w253) -> (w252:string[])
        n124 = case shown="True" w269 {
          tunnel: w249 -> [_ w295]
          tunnel: w247 -> [_ w296]
          frame False {
          }
          frame True {
            # "Channel 0"
            n125 = TDMS Write(0:w296, 9:w295) -> (4:w298:refnum<k34>, 15:w297:errorcluster)  [unwired: 4 in, 2 out]
            n126 = TDMS Close(8:w297, 11:w298) -> ()  [unwired: 2 out]
          }
        }
        n127 = case shown="True" w268 {
          tunnel: w250 -> [_ w291]
          tunnel: w246 -> [_ w292]
          frame False {
          }
          frame True {
            # "Channel 1"
            n128 = TDMS Write(0:w292, 9:w291) -> (4:w294:refnum<k34>, 15:w293:errorcluster)  [unwired: 4 in, 2 out]
            n129 = TDMS Close(8:w293, 11:w294) -> ()  [unwired: 2 out]
          }
        }
        n130 = case shown="True" w267 {
          tunnel: w251 -> [_ w287]
          tunnel: w245 -> [_ w288]
          frame False {
          }
          frame True {
            # "Channel 2"
            n131 = TDMS Write(0:w288, 9:w287) -> (4:w290:refnum<k34>, 15:w289:errorcluster)  [unwired: 4 in, 2 out]
            n132 = TDMS Close(8:w289, 11:w290) -> ()  [unwired: 2 out]
          }
        }
        n133 = case shown="True" w266 {
          tunnel: w252 -> [_ w283]
          tunnel: w244 -> [_ w284]
          frame False {
          }
          frame True {
            # "Channel 3"
            n134 = TDMS Write(0:w284, 9:w283) -> (4:w286:refnum<k34>, 15:w285:errorcluster)  [unwired: 4 in, 2 out]
            n135 = TDMS Close(8:w285, 11:w286) -> ()  [unwired: 2 out]
          }
        }
      }
      frame "Create File" {
        n136 = Unbundle(w313) -> ("Use Channel 0"=w312:bool, "Use Channel 1"=w311:bool, "Use Channel 2"=w310:bool, "Use Channel 3"=w309:bool)
        n137 = case shown="True" w312 {
          tunnel: [refnum<k34> refnum ("tdms file out") w336] -> w308
          frame False {
          }
          frame True {
            n138 = call "File Dialog4"("prompt"="Select or Create a File for Channel 0") -> ("selected path"=w339:path)  [unwired: 11 in, 3 out]
            n139 = TDMS Open(10:T8."create" ("operation (0:open)"), 11:w339) -> (3:w337:refnum<k34>)  [unwired: 5 in, 1 out]
            n140 = call "Header Data Creator.vi"("tdms file in"=w337, "Amplifier Metadata"="Amplifier Channel 3", "User Data"="User Data Channel 3") -> ("tdms file out"=w336:refnum<k34>)  [unwired: 6 in, 1 out]
          }
        }
        n141 = case shown="True" w311 {
          tunnel: [refnum<k34> refnum ("tdms file out") w342] -> w307
          frame False {
          }
          frame True {
            n142 = call "File Dialog3"("prompt"="Select or Create a File for Channel 1") -> ("selected path"=w347:path)  [unwired: 11 in, 3 out]
            n143 = TDMS Open(10:T8."create" ("operation (0:open)"), 11:w347) -> (3:w343:refnum<k34>)  [unwired: 5 in, 1 out]
            n144 = call "Header Data Creator.vi"("tdms file in"=w343, "Amplifier Metadata"="Amplifier Channel 2", "User Data"="User Data Channel 2") -> ("tdms file out"=w342:refnum<k34>)  [unwired: 6 in, 1 out]
          }
        }
        n145 = Get Date/Time String(date format (0)=enum16{"short", "long", "abbreviated"}."short") -> (date string=→"Date mm/dd/yy":string, time string=→"Start Time hr/min":string)  [unwired: 2 in]
        n146 = case shown="True" w310 {
          tunnel: [refnum<k34> refnum ("tdms file out") w318] -> w306
          frame False {
          }
          frame True {
            n147 = call "File Dialog2"("prompt"="Select or Create a File for Channel 2") -> ("selected path"=w323:path)  [unwired: 11 in, 3 out]
            n148 = TDMS Open(10:T8."create" ("operation (0:open)"), 11:w323) -> (3:w321:refnum<k34>)  [unwired: 5 in, 1 out]
            n149 = call "Header Data Creator.vi"("tdms file in"=w321, "Amplifier Metadata"="Amplifier Channel 1", "User Data"="User Data Channel 1") -> ("tdms file out"=w318:refnum<k34>)  [unwired: 6 in, 1 out]
          }
        }
        n150 = case shown="True" w309 {
          tunnel: [refnum<k34> refnum ("tdms file out") w328] -> w305
          frame False {
          }
          frame True {
            n151 = call "File Dialog"("prompt"="Select or Create a File for Channel 3") -> ("selected path"=w332:path)  [unwired: 11 in, 3 out]
            n152 = TDMS Open(10:T8."create" ("operation (0:open)"), 11:w332) -> (3:w329:refnum<k34>)  [unwired: 5 in, 1 out]
            n153 = call "Header Data Creator.vi"("tdms file in"=w329, "Amplifier Metadata"="Amplifier Channel 0", "User Data"="User Data Channel 0") -> ("tdms file out"=w328:refnum<k34>)  [unwired: 6 in, 1 out]
          }
        }
        n154 = Enqueue Element(queue=w302, element=Enum_State_Typedef."Record", error in (no error)=w301) -> ()  [unwired: 1 in, 3 out]
        n155 = Bundle("tdms file out"=w308, "tdms file out"=w307, "tdms file out"=w306, "tdms file out"=w305) -> (w304:T5)  [unwired: 1 in]
      }
      frame "Exit" {
      }
      frame "Record" {
        # "dt"
        n156 = property on="Sample Rate" class="DigNum (strict)"() -> ("Value"=w357:i32)  [unwired: 2 in, 2 out]
        n157 = Reciprocal(x=w357) -> (1/x=w356:dbl)
        n158 = Multiply(x=20, y=w356) -> (x*y=w367:dbl)
        n159 = call "TDMS Record.vi"("Data"=w353, "Input TDMS File Cluster"=w354, "In Use Cluster"=w355) -> ("Output TDMS File Cluster"=w352:T5)  [unwired: 8 in]
        n160 = call "Waveform Edit.vi"("Change in Time"=w367, "In Use Cluster"=w355, "New Data"=w353, "Old Data"=w366) -> ("Output Waveform Cluster"=w364:T11, "Output Decimated Data"=w365:dbl[][])  [unwired: 5 in, 1 out]
        n161 = Unbundle(w364) -> ("Waveform"=w363:waveform(dbl), "Waveform"=w362:waveform(dbl), "Waveform"=w361:waveform(dbl), "Waveform"=w360:waveform(dbl))
        n162 = Build Array(w363, w362, w361, w360) -> (w359:waveform(dbl)[])
        n163 = property on="Channel 0 Chart" class="WFChart (strict)"("Value"=w363) -> ()  [unwired: 2 in, 2 out]
        n164 = property on="Channel 1 Chart" class="WFChart (strict)"("Value"=w362) -> ()  [unwired: 2 in, 2 out]
        n165 = property on="Overview Chart" class="WFChart (strict)"("Value"=w359) -> ()  [unwired: 2 in, 2 out]
        n166 = property on="Channel 2 Chart" class="WFChart (strict)"("Value"=w361) -> ()  [unwired: 2 in, 2 out]
        n167 = property on="Channel 3 Chart" class="WFChart (strict)"("Value"=w360) -> ()  [unwired: 2 in, 2 out]
      }
    }
  }
